vi "arbitrary ICP waveform output.vi"() -> ()   [LabVIEW 2015]
uses:
  <vilib>/DAQmx/write.llb/DAQmx Write (Analog DBL 1Chan 1Samp).vi
  <vilib>/DAQmx/create/channels.llb/DAQmx Create Channel (AO-Voltage-Basic).vi
  <vilib>/DAQmx/miscellaneous.llb/DAQmx Fill In Error Info.vi
panel:
  out "Display Time":dbl
  out "test ICP input":cluster{i32[], dbl[]}(graph)
  out "Display Changing Pressure":dbl
  out "Supply Voltage":dbl
  in  "stop":bool
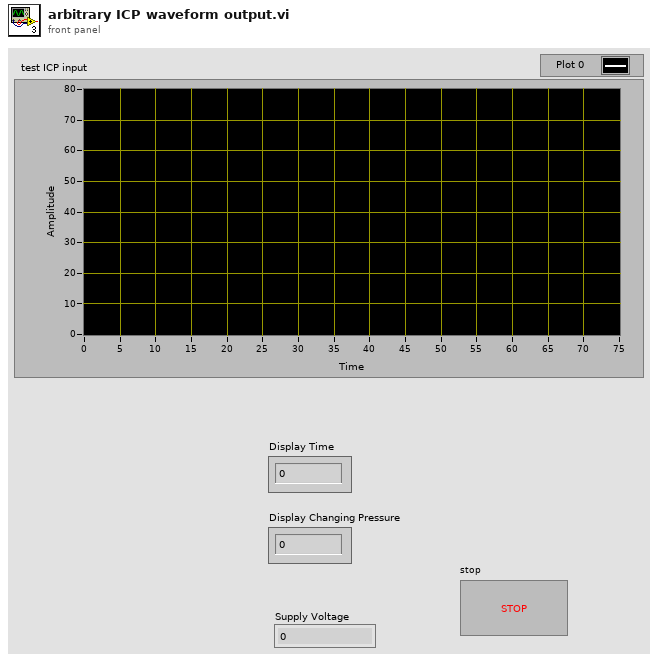
[diagram p1: front panel]
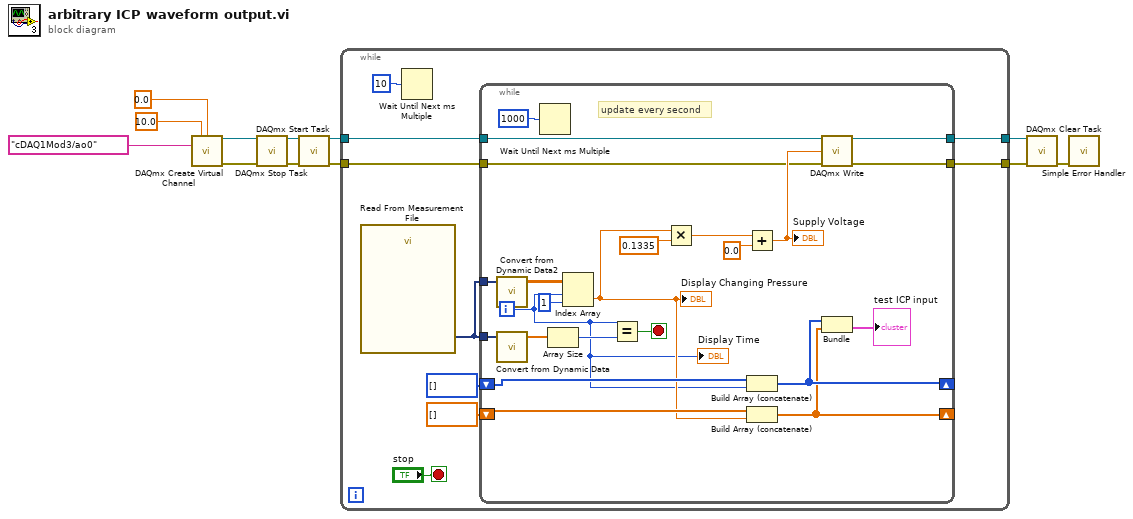
[diagram p0: block diagram]
diagram:
  n1 = call-poly <vilib>:"DAQmx Create Virtual Channel.vi"("maximum value"=10.0, "minimum value"=0.0, "physical channels"=tag "cDAQ1Mod3/ao0") -> ("task out"=w5:refnum<k21>, "error out"=w6:errorcluster)  [unwired: 11 in]
  n2 = call <vilib>:"DAQmx Stop Task.vi"("task/channels in"=w5, "error in"=w6) -> ("task out"=w3:refnum<k21>, "error out"=w4:errorcluster)  [unwired: 12 in]
  n3 = call <vilib>:"DAQmx Start Task.vi"("task/channels in"=w3, "error in"=w4) -> ("task out"=w11:refnum<k21>, "error out"=w12:errorcluster)  [unwired: 12 in]
  n4 = while {
    tunnel: [w16] -> w8
    tunnel: [w17] -> w9
    tunnel: w11 -> [w19]
    tunnel: w12 -> [w18]
    stop <- "stop" stop-if-true
    n5 = call "Read From Measurement File"() -> ("Signals"=w20:dynamicdata)  [unwired: 6 in, 5 out]
    n6 = Wait Until Next ms Multiple(millisecond multiple=u32 10) -> ()  [unwired: 1 out]
    n7 = while {
      tunnel: w20 -> [w44]
      tunnel: w20 -> [w39]
      tunnel: w19 -> [w33]
      tunnel: w18 -> [w32]
      tunnel: [w31] -> w17
      tunnel: [w30] -> w16
      shift-right: [w25] -> _
      shift-left: i32[] [] -> [w28]
      shift-right: [w24] -> _
      shift-left: dbl[] [] -> [w27]
      i -> [w22]
      stop <- w42 stop-if-true
      # "update every second"
      n8 = call "Convert from Dynamic Data2"("Dynamic Data Type"=w39) -> ("Array"=w40:dbl[][])  [unwired: 3 in]
      n9 = call "Convert from Dynamic Data"("Dynamic Data Type"=w44) -> ("Array"=w43:dbl[])  [unwired: 3 in]
      n10 = Wait Until Next ms Multiple(millisecond multiple=u32 1000) -> ()  [unwired: 1 out]
      n11 = Array Size(array=w43) -> (size(s)=w23:i32)
      n12 = Index Array(array=w40, index (row)=w22, index (col)=1) -> (element=w26:dbl)
      "Display Changing Pressure" <- w26
      n13 = Equal?(x=w22, y=w23) -> (x = y?=w42:bool)
      n14 = Multiply(x=w26, y=0.1335 ("x")) -> (x*y=w35:dbl)
      n15 = Add(x=w35, y=0.0) -> (x+y=w34:dbl)
      "Supply Voltage" <- w34
      n16 = Build Array (concatenate)(w28, w22) -> (w25:i32[])
      n17 = Build Array (concatenate)(w27, w26) -> (w24:dbl[])
      n18 = call-poly <vilib>:"DAQmx Write.vi"("task/channels in"=w33, "data"=w34, "error in"=w32) -> ("task out"=w30:refnum<k21>, "error out"=w31:errorcluster)  [unwired: 10 in, 1 out]
      n19 = Bundle(w25, w24) -> (→"test ICP input":cluster{i32[], dbl[]})  [unwired: 1 in]
      "Display Time" <- w22
    }
  }
  n20 = call <vilib>:"DAQmx Clear Task.vi"("task in"=w8, "error in"=w9) -> ("error out"=w10:errorcluster)  [unwired: 13 in]
  n21 = call <vilib>:"Simple Error Handler.vi"("error in (no error)"=w10) -> ()  [unwired: 4 in, 5 out]
